vi "Parse Response.vi"(8 "error in (no error)":errorcluster, 10 "{JSON} Response":string, 11 "JSON-RPC in":refnum<class "JSON-RPC.lvclass">) -> (0 "error out":errorcluster, 1 "Array":bool[](array[boolean]), 2 "results":string[](array[string]), 3 "JSON-RPC out":refnum<class "JSON-RPC.lvclass">)   [LabVIEW 2019, in "JSON-RPC.lvclass"]
uses:
  JSON-RPC.lvclass
  JSON-RPC.lvclass/JSON-RPC.ctl
  private/Parse Response-JSONtext.vi/7ce7fba8-9f44-478d-b6cb-b571ff29f2f5.vi
  private/Parse Response-JSONtext.vi/8c905beb-ab4c-49e3-b5c6-2c663b7b30d7.vi
  private/Parse Response-JSONtext.vi/fce5892e-0c40-47e1-88e0-6c122aadefe2.vi
  <vilib>/JDP Science/JSONtext/Find Item.vi
  <vilib>/JDP Science/JSONtext/String Subset.vi
  <vilib>/JDP Science/JSONtext/Get all Object Items.vi
  <vilib>/JDP Science/JSONtext/Parsing/Parse Full Path or Item Name.vi
  <vilib>/JDP Science/JSONtext/Next JSON Value.vi
  <vilib>/JDP Science/JSONtext/support/Error Cluster From Code.vi
  <vilib>/JDP Science/JSONtext/Offset/Find Item Locations by Path.vi
  <vilib>/JDP Science/JSONtext/JSON text to Variant.vi
  <vilib>/Utility/error.llb/Error Cluster From Error Code.vi
  <vilib>/JDP Science/JSONtext/LVClass Serializer/JSONtext LVClass Serializer.lvclass
  <vilib>/JDP Science/JSONtext/JSONtext.lvlib
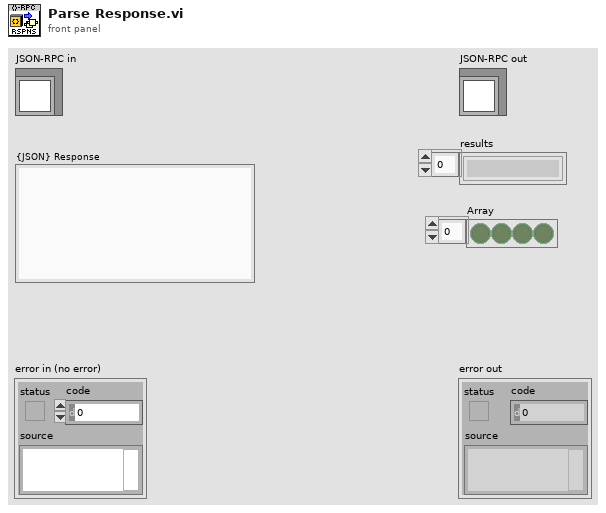
[diagram p1: front panel]
types:
  T1 = typedef "JSONtext.lvlib/JSON Value Type.ctl" = enum16{"Not a JSON Value", "JSON Object", "JSON Array", "String", "Number", "true", "false", "null"}
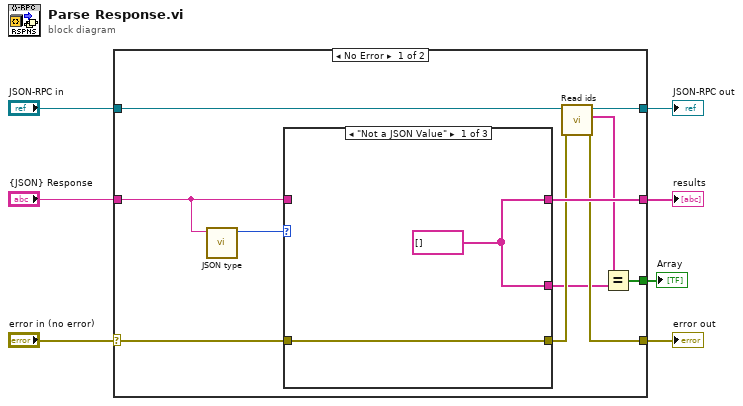
[diagram p0: block diagram]
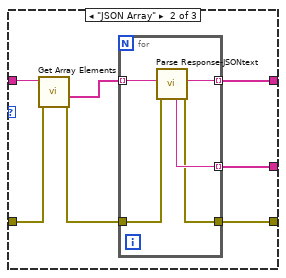
[diagram p2: hidden frame]
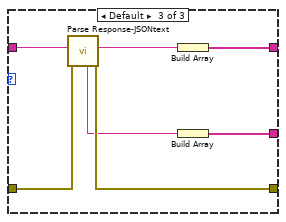
[diagram p3: hidden frame]
diagram:
  n1 = case shown="No Error" "error in (no error)" {
    selector: "error in (no error)" -> [w16 w41]
    tunnel: [w11 w41] -> w6
    tunnel: "JSON-RPC in" -> [w13 w40]
    tunnel: "{JSON} Response" -> [w17 _]
    tunnel: [w14 w40] -> w3
    tunnel: [w15 _] -> w2
    tunnel: [w8 _] -> w1
    frame No Error {
      n2 = call <vilib>:"JSON type.vi"("JSON"=w17) -> ("JSON Value Type"=w18:T1)  [unwired: 9 in, 1 out]
      n3 = case shown="\"Not a JSON Value\"" w18 {
        tunnel: w16 -> [w20 w24 w36]
        tunnel: [w20 w27 w35] -> w12
        tunnel: w17 -> [_ w25 w37]
        tunnel: [w19 w26 w39] -> w15
        tunnel: [w19 w22 w38] -> w9
        frame "Not a JSON Value" {
          w19 = string[] []
        }
        frame "JSON Array" {
          n4 = call <vilib>:"Get Array Elements.vi"("error in (no error)"=w24, "JSON"=w25) -> ("error out"=w21:errorcluster, "<JSON>"=w23:string[])  [unwired: 7 in, 1 out]
          n5 = for {
            tunnel: w23 -> [w32] mode=indexing
            tunnel: [w30] -> w26 mode=indexing
            tunnel: [w29] -> w22 mode=indexing
            tunnel: w21 -> [w31]
            tunnel: [w28] -> w27
            n6 = call "Parse Response-JSONtext.vi"("error in (no error)"=w31, "{JSON} Response"=w32) -> ("error out"=w28:errorcluster, "result"=w30:string, "id"=w29:string)  [unwired: 7 in]
          }
        }
        frame Default {
          n7 = call "Parse Response-JSONtext.vi"("error in (no error)"=w36, "{JSON} Response"=w37) -> ("error out"=w35:errorcluster, "result"=w33:string, "id"=w34:string)  [unwired: 7 in]
          n8 = Build Array(w33) -> (w39:string[])
          n9 = Build Array(w34) -> (w38:string[])
        }
      }
      n10 = call "Read ids.vi"("error in (no error)"=w12, "JSON-RPC in"=w13) -> ("error out"=w11:errorcluster, "ids"=w10:string[], "JSON-RPC out"=w14:refnum<class "JSON-RPC.lvclass">)  [unwired: 7 in]
      n11 = Equal?(x=w10, y=w9) -> (x = y?=w8:bool[])
    }
    frame Error {
    }
  }
  "error out" <- w6
  "JSON-RPC out" <- w3
  "results" <- w2
  "Array" <- w1
